vi "RNN_full_iteration_demo.vi"(0 "_vocab size":i32=3, 1 "learning_rate":dbl=0.1, 5 "_inputs":i32[](array[numeric])=[1], 7 "targets":i64[](array[numeric])=[0], 9 "_hprev":T1=[[0.0], [0.0]], 11 "_params":T2={"Wxh"=[[0.578129, 2.569937, -0.0219857], [-2.46959, 0.027262, 2.449614362]], "Whh"=[[-1.3996, 0.961745], [0.364566, -0.477064]], "bh"=[[0.535351], [-1.985987]], "Why"=[[-0.658616, 0.764692], [-1.7789986, 0.388036], [-0.130912, -0.333988]], "by"=[[-0.528417], [-0.44032], [-0.8844819]]} {"Wxh" format="%_8f"; "Whh" format="%_8f"; "bh" format="%_8f"; "Why" format="%_8f"; "by" format="%_8f"}) -> (4 "h_latest":T1=[[0.9959918876590693], [-0.9609924209716473]], 6 "dParams_":T3={"dWxh"=[[0.0, 0.0019862373697962215, 0.0], [0.0, -0.06118825535684556, 0.0]], "dWhh"=[[0.0, 0.0], [0.0, 0.0]], "dbh"=[[0.0019862373697962215], [-0.06118825535684556]], "dWhy"=[[-0.7935213511320954, 0.7656367624734651], [0.10403870131705772, -0.10038274878765777], [0.6894826498150377, -0.6652540136858074]], "dby"=[[-0.796714673045329], [0.10445737822381787], [0.6922572948215111]]} {"dWxh" format="%_8f"; "dWhh" format="%_8f"; "dbh" format="%_8f"; "dWhy" format="%_8f"; "dby" format="%_8f"}, 15 "params_":T2={"Wxh"=[[0.578129, 2.470063497819347, -0.0219857], [-2.46959, 0.1272618664533515, 2.449614362]], "Whh"=[[-1.3996, 0.961745], [0.364566, -0.477064]], "bh"=[[0.43547749781934725], [-1.8859871335466485]], "Why"=[[-0.5586160007940589, 0.6646920008529518], [-1.8789985538066074, 0.48803595038059944], [-0.23091199894822387, -0.2339880011297829]], "by"=[[-0.4284170007877064], [-0.5403199541761617], [-0.9844818989566383]]} {"Wxh" format="%_8f"; "Whh" format="%_8f"; "bh" format="%_8f"; "Why" format="%_8f"; "by" format="%_8f"})   [LabVIEW 2014]
uses:
  <vilib>/Analysis/Matrix/Datatypes/RealMatrix.ctl
  <vilib>/Analysis/Matrix/NI_Matrix.lvlib
panel:
  out "Losses":dbl[](array[numeric]) format="%_8f"
  out "Total Loss":dbl format="%_8f"
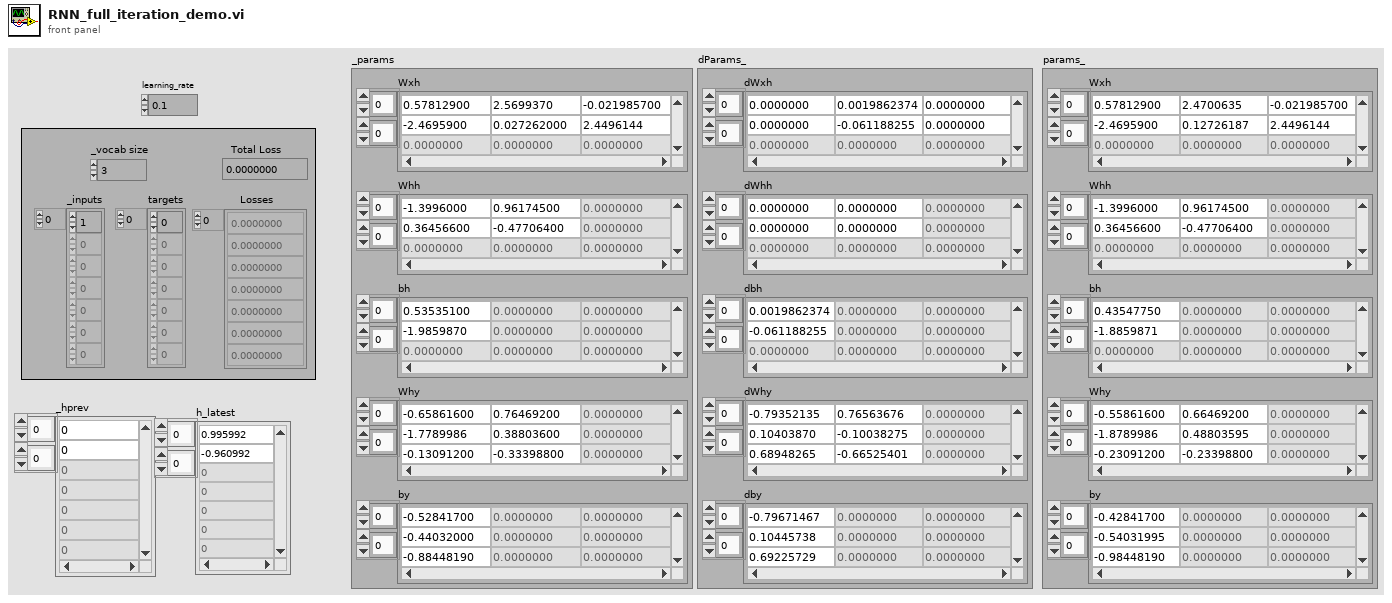
[diagram p1: front panel]
types:
  T1 = typedef "NI_Matrix.lvlib/RealMatrix.ctl" = dbl[][]
  T2 = cluster{"Wxh":T1, "Whh":T1, "bh":T1, "Why":T1, "by":T1}
  T3 = cluster{"dWxh":T1, "dWhh":T1, "dbh":T1, "dWhy":T1, "dby":T1}
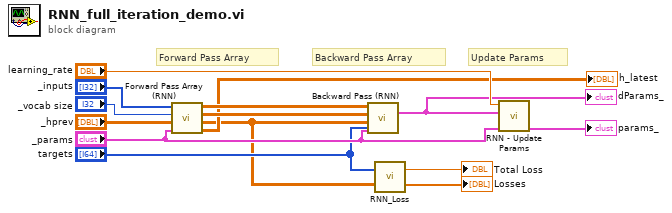
[diagram p0: block diagram]
diagram:
  # "Update Params"
  # "Backward Pass Array"
  # "Forward Pass Array"
  n1 = call "Forward Pass Array (RNN).vi"("inputs"="_inputs", "vocab size"="_vocab size", "hprev"="_hprev", "params"="_params") -> ("xs"=w13:dbl[][][], "hs"=w14:dbl[][][], "ps"=w1:dbl[][][], "h_latest"=→"h_latest":T1)  [unwired: 3 in]
  n2 = call "Backward Pass (RNN).vi"("xs"=w13, "hs"=w14, "ps"=w1, "targets"="targets", "params"="_params") -> ("dParams_"=w7:T3)  [unwired: 10 in]
  "dParams_" <- w7
  n3 = call "RNN_Loss.vi"("targets"="targets", "ps"=w1) -> ("Loss (total)"=→"Total Loss":dbl, "Loss Array"=→"Losses":dbl[])  [unwired: 16 in]
  n4 = call "RNN - Update Params.vi"("learning_rate"="learning_rate", "dParams"=w7, "_params"="_params") -> ("params_"=→"params_":T2)  [unwired: 5 in]
